vi "Read List Table Name.vi"(8 "error in (no error)":errorcluster, 11 "Settings in":refnum<class "Settings.lvclass">) -> (0 "error out":errorcluster, 2 "List Table Name":refnum<vi>, 3 "Settings out":refnum<class "Settings.lvclass">)   [LabVIEW 2023, in "GUI.lvlib" / "Settings.lvlib" / "Settings.lvclass"]
uses:
  Settings.lvclass
  Settings.lvclass/Settings.ctl
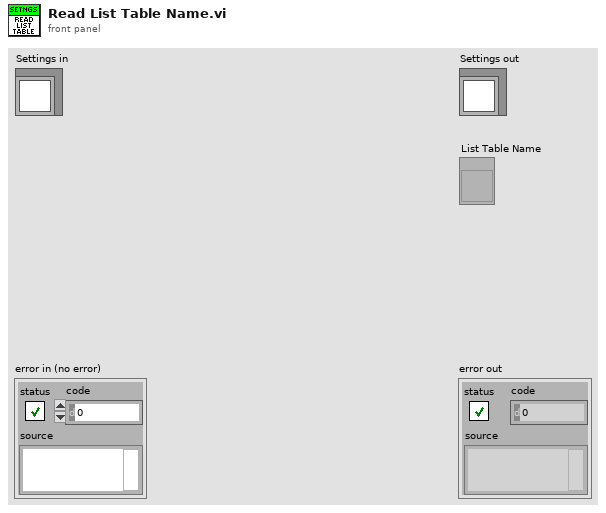
[diagram p1: front panel]
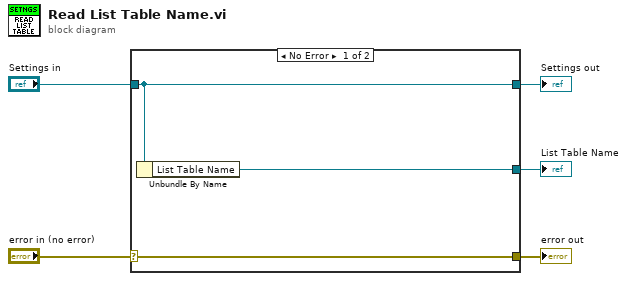
[diagram p0: block diagram]
diagram:
  n1 = case shown="No Error" "error in (no error)" {
    selector: "error in (no error)" -> [w8 w9]
    tunnel: [w8 w9] -> w4
    tunnel: [w7 w10] -> w2
    tunnel: "Settings in" -> [w7 w10]
    tunnel: [w6 _] -> w1
    frame No Error {
      n2 = Unbundle By Name(w7) -> ("List Table Name"=w6:refnum<vi>)
    }
    frame Error {
    }
  }
  "error out" <- w4
  "Settings out" <- w2
  "List Table Name" <- w1
